vi "ScanPoints.vi"(6 "NumPoints":i32, 7 "NumberSweeps":i32, 8 "UpdatesPerPoint":u32, 9 "ClockPause":u32=40, 10 "WriteSize":enum16{"1", "2", "4"}(ring), 11 "Point Delay(uSec)":u32 caption="Point Delay (uSec)") -> ()   [LabVIEW 2009]
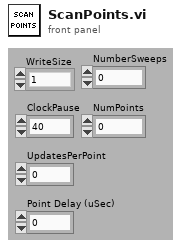
[diagram p1: front panel]
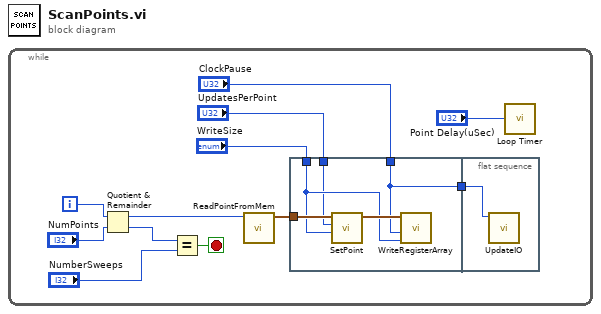
[diagram p0: block diagram]
diagram:
  n1 = while {
    i -> [w7]
    stop <- w3 stop-if-true
    n2 = Quotient & Remainder(x=w7, y="NumPoints") -> (x-y*floor(x/y)=w2:i32, floor(x/y)=w5:i32)
    n3 = Equal?(x=w5, y="NumberSweeps") -> (x = y?=w3:bool)
    n4 = call "ReadPointFromMem.vi"("PointNum"=w2) -> ("Point"=w1:cluster{"X":i32, "Y":i32, "Z":i32})  [unwired: 10 in]
    n5 = flat-sequence {
      tunnel: w1 -> [w17]
      tunnel: "WriteSize" -> [w15]
      tunnel: "UpdatesPerPoint" -> [w14]
      tunnel: "ClockPause" -> [w13]
      tunnel: [w13] -> w12
      tunnel: w12 -> [w18]
      frame #0 {
        n6 = call "SetPoint.vi"("WriteSize"=w15, "UpdatesPerPoint"=w14, "Point"=w17) -> ("Register Writes"=w16:cluster{"Address":u8, "Value":u32}[])  [unwired: 7 in, 1 out]
        n7 = call "WriteRegisterArray.vi"("WriteSize"=w15, "ClockPause"=w13, "Register  Values"=w16) -> ()  [unwired: 9 in]
      }
      frame #1 {
        n8 = call "UpdateIO.vi"("Count(ticks)"=w18) -> ()  [unwired: 11 in]
      }
    }
    n9 = call "Loop Timer"("Count(uSec)"="Point Delay(uSec)") -> ()  [unwired: 1 out]
  }
